vi "Get Channel Waveform Path.vi"(0 "Target":string, 1 "Channel":string) -> (7 "Topic":string)   [LabVIEW 2016]
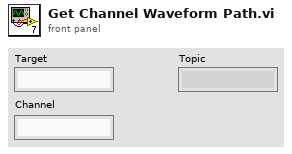
[diagram p1: front panel]
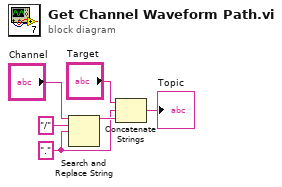
[diagram p0: block diagram]
diagram:
  w4 = "." ("replace string (\"\")")
  n1 = Search and Replace String(input string="Channel", search string="/", replace string=w4) -> (result string=w5:string)  [unwired: 5 in, 3 out]
  n2 = Concatenate Strings("Target", w4, w5) -> (→"Topic":string)
